vi "Send Close Shutter.vi"(7 "Message Priority (Normal)":T2=enum."Normal", 8 "error in (no error)":errorcluster, 10 "Shutter to Close":T1=enum."Cy3 (532 nm)", 11 "Message Enqueuer":refnum<class "Message Enqueuer.lvclass">) -> (0 "error out":errorcluster, 3 "Message Enqueuer out":refnum<class "Message Enqueuer.lvclass">)   [LabVIEW 2015, in "Uniblitz Shutter.lvlib" / "Close Shutter Msg.lvclass"]
doc: "This VI sends the message to an actor."
uses:
  Close Shutter Msg.lvclass
  <vilib>/ActorFramework/Message Enqueuer/Message Enqueuer.lvclass
  <vilib>/ActorFramework/Message Enqueuer/Message Priority.ctl
  Resources/Type Defs/Excitation.ctl
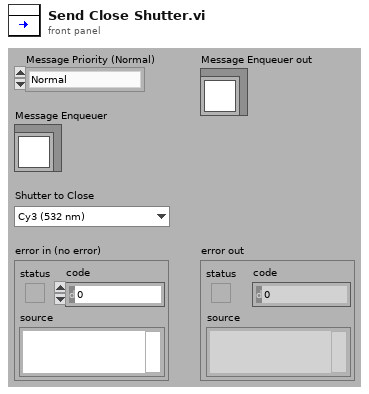
[diagram p1: front panel]
types:
  T1 = typedef "Excitation.ctl" = enum16{"Cy2 (473 nm)", "Cy3 (532 nm)", "Cy5 (639 nm)", "Cy7 (730 nm)"}
  T2 = typedef "Actor Framework.lvlib/Message Enqueuer.lvclass/Message Priority.ctl" = enum16{"Low", "Normal", "High"}
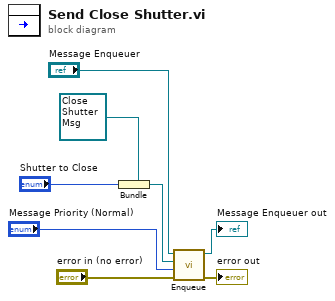
[diagram p0: block diagram]
diagram:
  n1 = Bundle(cluster=refnum<class "Close Shutter Msg.lvclass"> refnum ("Object"), "Shutter to Close") -> (w4:refnum<class "Close Shutter Msg.lvclass">)
  n2 = call <vilib>:"Enqueue.vi"("error in (no error)"="error in (no error)", "Message Priority (Normal)"="Message Priority (Normal)", "Message"=w4, "Message Enqueuer in"="Message Enqueuer") -> ("error out"=→"error out":errorcluster, "Message Enqueuer out"=→"Message Enqueuer out":refnum<class "Message Enqueuer.lvclass">)  [unwired: 6 in]
